vi "merge_Collect Numeric Array.vi"   [LabVIEW 2017]
doc: "Accumulates numeric input elements when <B>enable</B> is TRUE. The <B>collected data</B> array contains the collection of input elements. If <B>collected data</B> reaches the capacity you specify using the <B>array size</B> input, the function block discards additional <B>input</B> values until you clear the function block by setting the <B>reset</B> input to TRUE."
uses:
  <vilib>/functionblocks/FB Core/FB Core.xnode
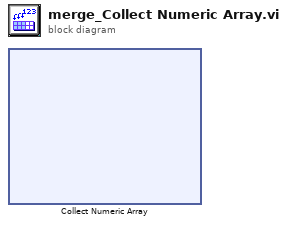
[diagram p0: block diagram]
diagram:
  n1 = xnode "Collect Numeric Array"() -> ()  [unwired: 5 in, 4 out]
